vi "MGCC_StaEst_initial_1.vi"() -> ()   [LabVIEW 2016]
uses:
  <vilib>/imath/engines/lvmath2/RunTimeEngine/RunTimeType/NIMS_RunTimeType_From StrictType (excl LVString).vi
  <vilib>/imath/engines/lvmath2/RunTimeEngine/Struct/NIMS_StructSetField.vi
  <vilib>/imath/engines/lvmath2/RunTimeEngine/Struct/NIMS_StructGetField.vi
  <vilib>/imath/engines/lvmath2/RunTimeEngine/RunTimeType/NIMS_RunTimeType_To Numeric.vi
  <vilib>/imath/engines/lvmath2/RunTimeEngine/BuiltInFunctions/imag/NIMS_imag(Complex).vi
  <vilib>/imath/engines/lvmath2/RunTimeEngine/NodeEndStatement/NIMS_NodeEndStatement_Output.vi
  <vilib>/imath/engines/lvmath2/RunTimeEngine/ErrorHandling/NIMS_Finalize Error.vi
panel:
  out "error out":errorcluster
  out "str_MGCC_MdlMgmt_Feeder":T1
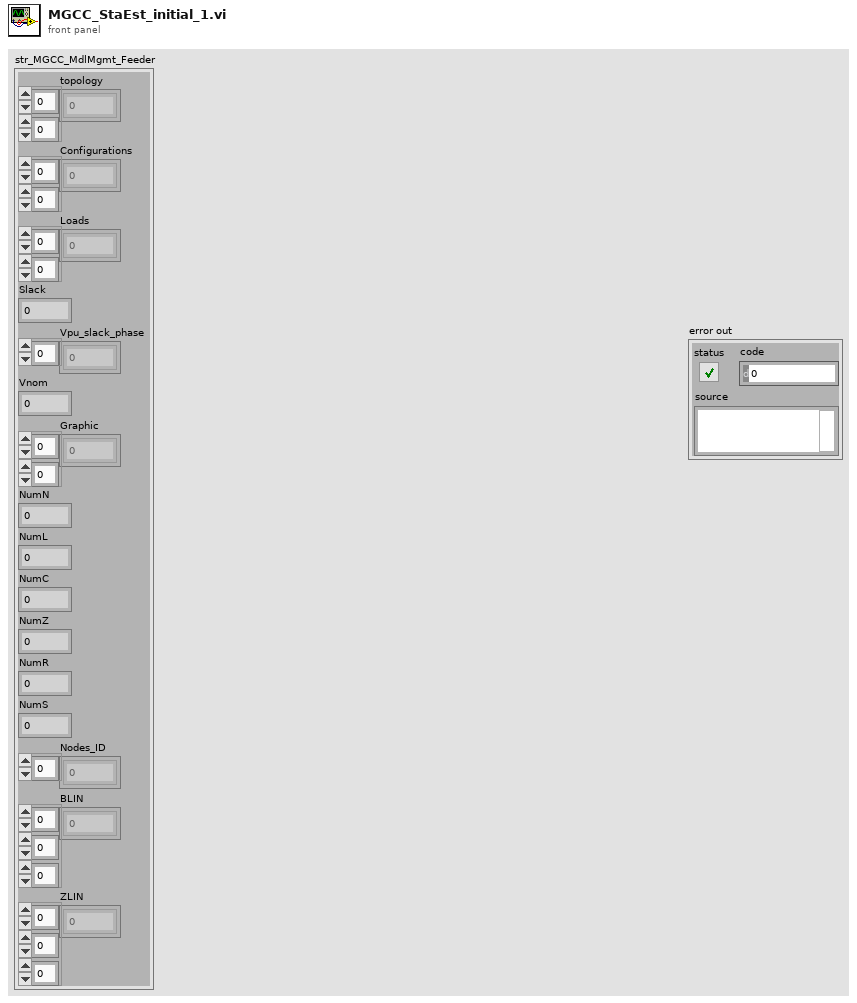
[diagram p1: front panel]
types:
  T1 = cluster{"topology":dbl[][], "Configurations":dbl[][], "Loads":dbl[][], "Slack":dbl, "Vpu_slack_phase":cdb[], "Vnom":dbl, "Graphic":dbl[][], "NumN":dbl, "NumL":dbl, "NumC":dbl, "NumZ":dbl, "NumR":dbl, "NumS":dbl, "Nodes_ID":dbl[], "BLIN":cdb[][][], "ZLIN":cdb[][][]}
  T2 = cluster{"VOL":cdb[][], "PN":dbl[][], "QN":dbl[][], "IN":dbl[][], "Ve":dbl[][], "Vf":dbl[][], "VN":dbl[][], "AN":dbl[][]}
  T3 = cluster{"Sbase":dbl, "Vbase":dbl, "Ibase":dbl, "Ybase":dbl}
  T4 = cluster{"Node":dbl, "Line":dbl, "StateVar":i32, "Zeroinj":i32}
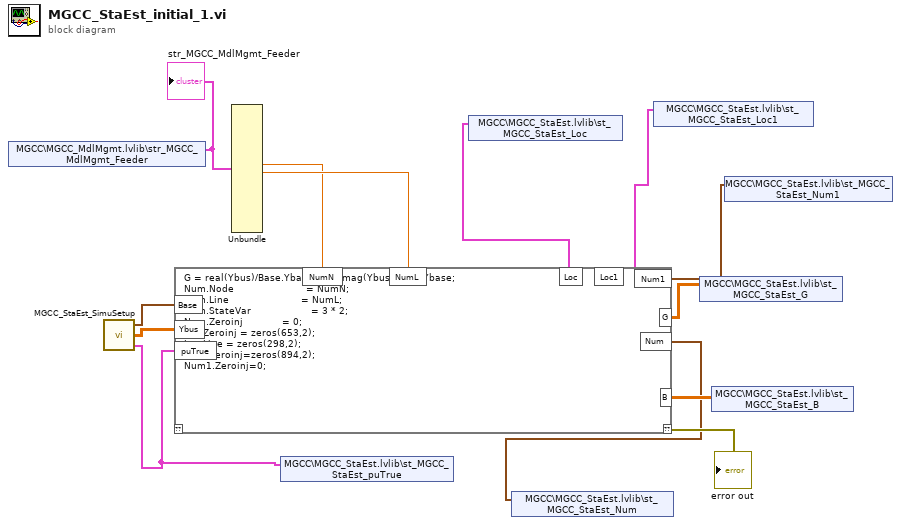
[diagram p0: block diagram]
diagram:
  n1 = shared-variable "MGCC\\MGCC_MdlMgmt.lvlib\\str_MGCC_MdlMgmt_Feeder"() -> (w11:T1)  [unwired: 1 in, 1 out]
  "str_MGCC_MdlMgmt_Feeder" <- w11
  n2 = call "MGCC_StaEst_SimuSetup.vi"() -> ("puTrue"=w3:T2, "Ybus"=w12:cdb[][], "Base"=w13:T3)  [unwired: 3 in]
  n3 = Unbundle(w11) -> ("NumN"=w9:dbl, "NumL"=w10:dbl)  [unwired: 14 out]
  n4 = mathscript code="G = real(Ybus)/Base.Ybase; B = imag(Ybus)/Base.Ybase;\nNum.Node                        = NumN;\nNum.Line                        = NumL;\nNum.StateVar                    = 3 * 2;  \nNum.Zeroinj             = 0;\nLoc.Zeroinj = zeros(653,2);\nLoc.Line = zeros(298,2);\nLoc1.Zeroinj=zeros(894,2);\nNum1.Zeroinj=0;"("Base"=w13, "Ybus"=w12, "puTrue"=w3, "NumN"=w9, "NumL"=w10) -> ("??"=→"error out":errorcluster, "G"=w7:dbl[][], "Num"=w5:T4, "Num1"=w1:cluster{"Zeroinj":i32}, "Loc"=w4:cluster{"Zeroinj":i32[][], "Line":i32[][]}, "Loc1"=w2:cluster{"Zeroinj":i32[][]}, "B"=w8:dbl[][])  [unwired: 1 in]
  n5 = shared-variable "MGCC\\MGCC_StaEst.lvlib\\st_MGCC_StaEst_puTrue"(w3) -> ()  [unwired: 1 in, 1 out]
  n6 = shared-variable "MGCC\\MGCC_StaEst.lvlib\\st_MGCC_StaEst_Loc"(w4) -> ()  [unwired: 1 in, 1 out]
  n7 = shared-variable "MGCC\\MGCC_StaEst.lvlib\\st_MGCC_StaEst_Num"(w5) -> ()  [unwired: 1 in, 1 out]
  n8 = shared-variable "MGCC\\MGCC_StaEst.lvlib\\st_MGCC_StaEst_Loc1"(w2) -> ()  [unwired: 1 in, 1 out]
  n9 = shared-variable "MGCC\\MGCC_StaEst.lvlib\\st_MGCC_StaEst_G"(w7) -> ()  [unwired: 1 in, 1 out]
  n10 = shared-variable "MGCC\\MGCC_StaEst.lvlib\\st_MGCC_StaEst_B"(w8) -> ()  [unwired: 1 in, 1 out]
  n11 = shared-variable "MGCC\\MGCC_StaEst.lvlib\\st_MGCC_StaEst_Num1"(w1) -> ()  [unwired: 1 in, 1 out]
